vi "Plot_XY_data.vi"(0 "Channel Values":string[][](array[string]), 1 "Ordinate Strings":string[](array[string]), 2 "Swap color and symbol":i32, 3 "Error Bar Chs":i32[](array[numeric])=[11], 5 "Accept Array":bool[][](array[boolean]), 7 "Filter 1 Strings":string[](array[string]), 9 "Filter 2 Strings":string[](array[string]), 11 "Ordinate":i32[](array[numeric])=[11], 12 "Absisca":u16, 13 "Transpose":bool) -> (15 "Accept Array Out":bool[][](array[boolean]))   [LabVIEW 2015]
uses:
  Results_plotter_Global.vi
panel:
  out "Colour Array":u32[][](array[colorbox])=[[26112, 39168, 52224, 65280, 65433], [153, 13311, 26367, 52479, 65535], [16711680, 16724838, 16737894, 16737945, 16751103], [16776960, 16777062, 16777113, 16777164, 16777215], [65280, 65280, 65280, 65280, 65280], [65280, 65280, 65280, 65280, 102]]
  out "Point Choice":u8[](array[numeric])=[10, 1, 11, 15, 5, 13, 2, 14]
  in  "Index Filter2":i32
  in  "Index Filter1":i32
  in  "Index Ordinate":i32
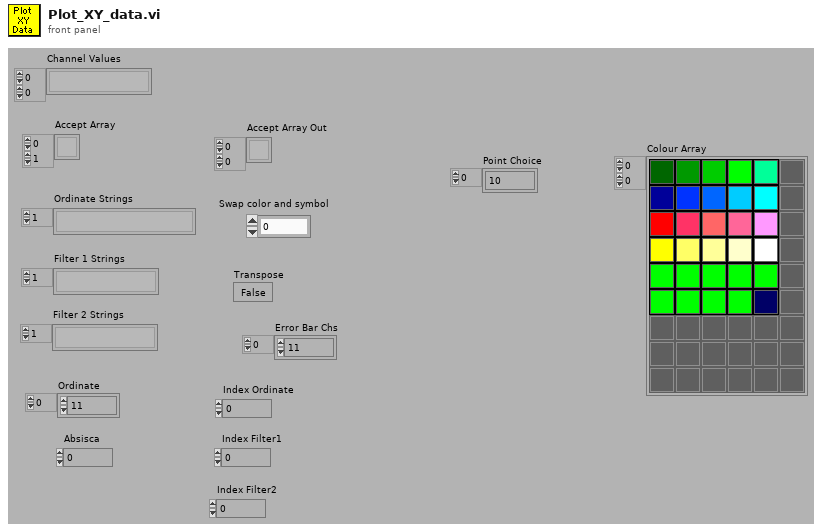
[diagram p1: front panel]
types:
  T1 = cluster{"Plot Color":u32, "Plot Interpolation":u8, "Point Style":u8, "Line Style":u8, "Fill/Pt. Color":u32, "Line Width":u8, "Bar Plot Style":u8, "Fill To":i16}
  T2 = cluster{"Averaged Values":dbl[], "Positions":dbl[]}[]
  T3 = cluster{"Plot Color":u32, "Plot Interpolation":u8, "Point Style":u8, "Line Style":u8, "Fill/Pt. Color":u32, "Line Width":u8, "Bar Plot Style":u8, "Fill To":i16}[]
  T4 = cluster{"Positions":dbl[], "Averaged Values":dbl[]}
  T5 = cluster{"Averaged Values":dbl[], "Positions":dbl[]}
  T6 = enum16{"Points", "StepLeft", "Line", "StepRight", "StepCentre", "StepEdge"}
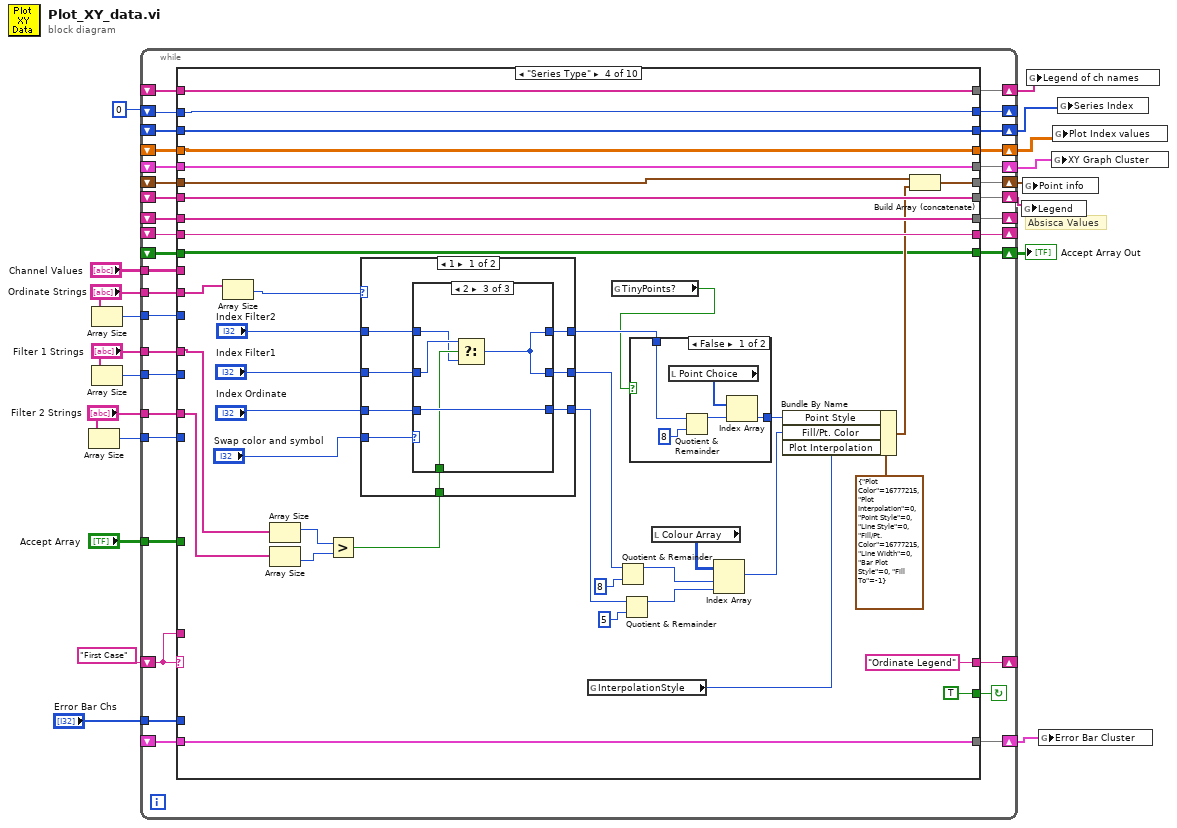
[diagram p0: block diagram]
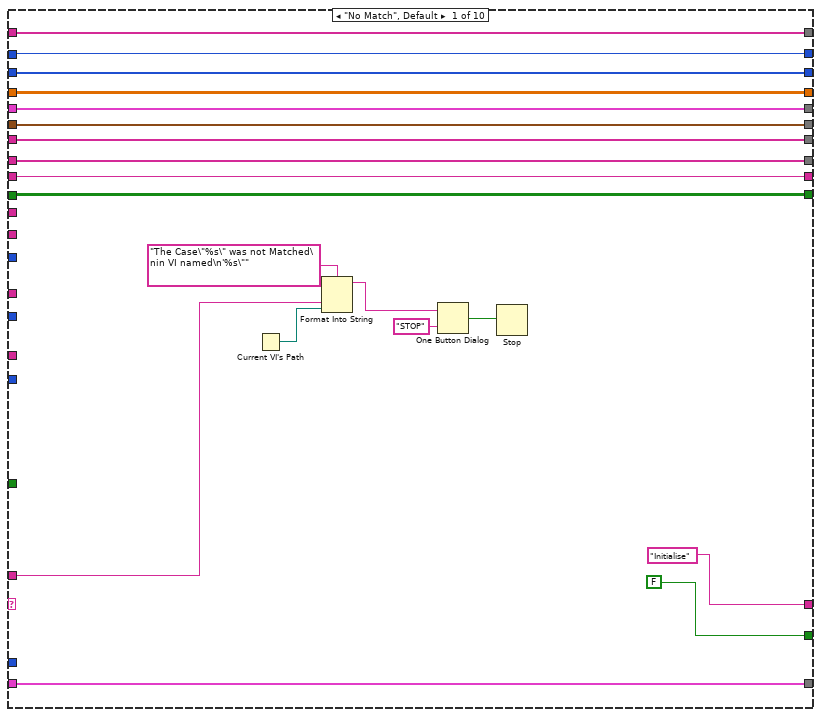
[diagram p2: hidden frame]
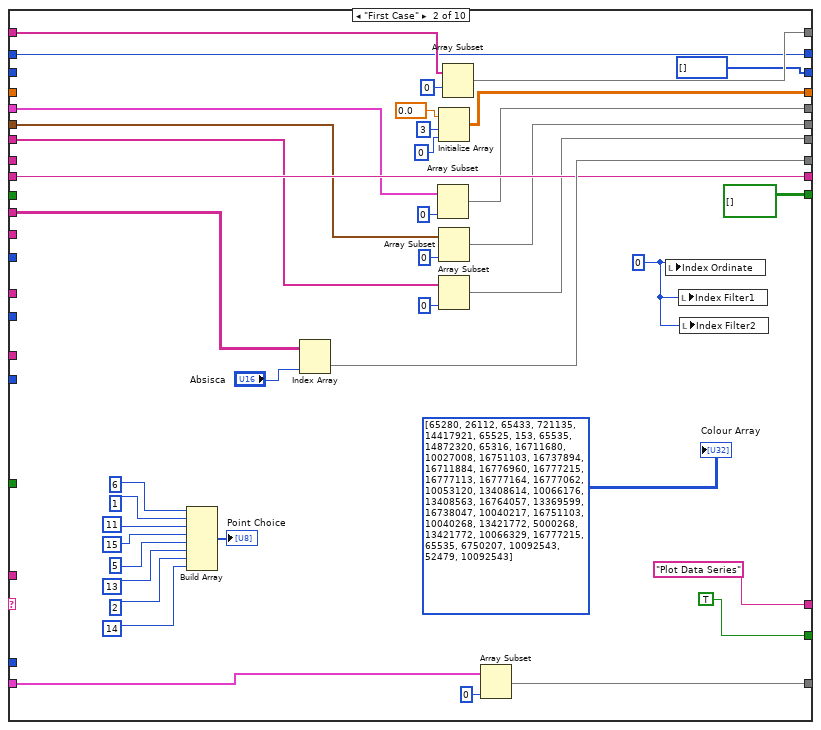
[diagram p3: hidden frame]
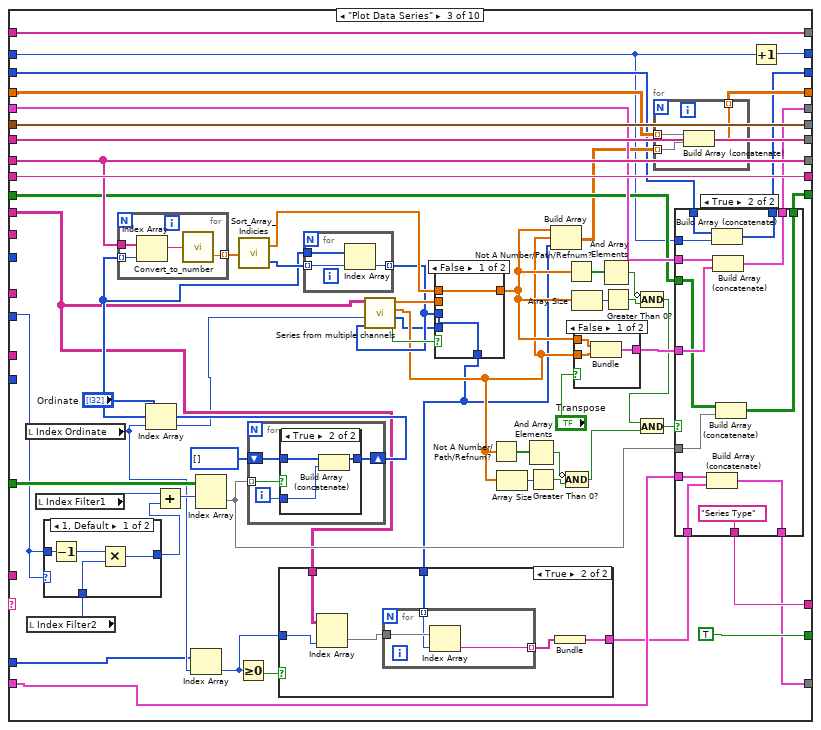
[diagram p4: hidden frame]
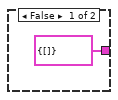
[diagram p6: hidden frame]
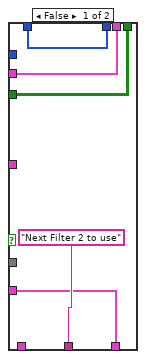
[diagram p8: hidden frame]
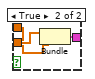
[diagram p9: hidden frame]
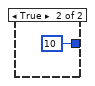
[diagram p11: hidden frame]
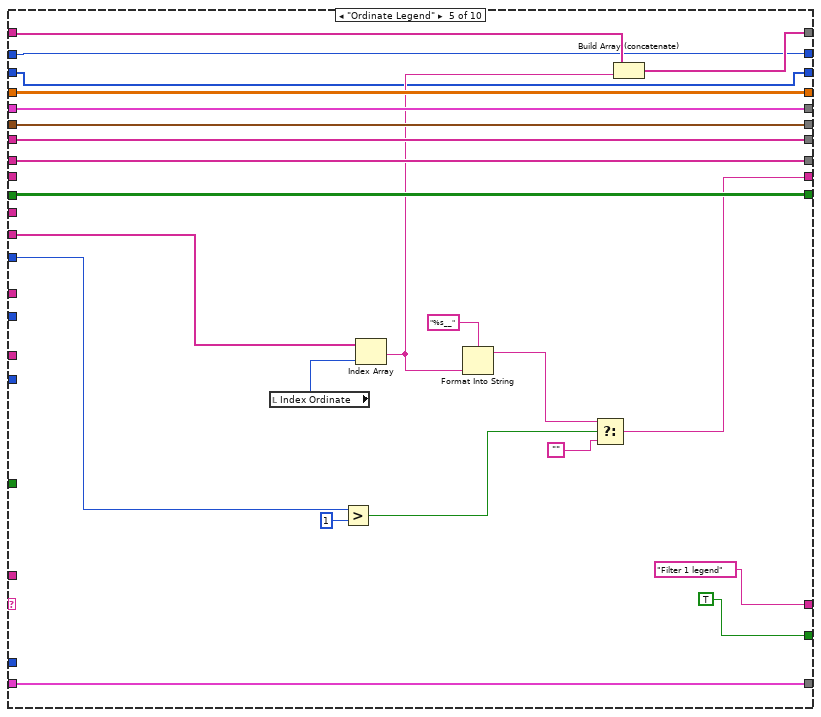
[diagram p20: hidden frame]
diagram:
  # "Absisca Values"
  n1 = Array Size(array="Filter 2 Strings") -> (size(s)=w12:i32)
  n2 = Array Size(array="Ordinate Strings") -> (size(s)=w13:i32)
  n3 = Array Size(array="Filter 1 Strings") -> (size(s)=w11:i32)
  n4 = while {
    shift-left: _ -> [w32]
    shift-right: [w31] -> w10
    tunnel: w11 -> [w33]
    tunnel: w12 -> [w34]
    tunnel: w13 -> [w35]
    tunnel: "Filter 1 Strings" -> [w36]
    tunnel: "Filter 2 Strings" -> [w37]
    tunnel: "Ordinate Strings" -> [w38]
    tunnel: "Accept Array" -> [w39]
    tunnel: "Channel Values" -> [w40]
    shift-left: _ -> [w41]
    shift-right: [w42] -> _
    shift-left: _ -> [w43]
    shift-right: [w44] -> _
    shift-left: _ -> [w46]
    shift-right: [w45] -> w7
    shift-left: _ -> [w48]
    shift-right: [w47] -> w8
    shift-left: _ -> [w50]
    shift-right: [w49] -> w6
    shift-left: "First Case" -> [w51]
    shift-right: [w52] -> _
    shift-right: [w29] -> w9
    shift-left: _ -> [w30]
    shift-right: [w28] -> w5
    shift-left: _ -> [w27]
    tunnel: "Error Bar Chs" -> [w26]
    shift-right: [w24] -> w3
    shift-left: _ -> [w25]
    shift-right: [w22] -> _
    shift-left: 0 -> [w23]
    shift-right: [w20] -> w1
    shift-left: _ -> [w21]
    stop <- w53 continue-if-true
    n5 = case shown="\"Series Type\"" w51 {
      tunnel: [FALSE TRUE TRUE TRUE TRUE TRUE TRUE TRUE TRUE w473] -> w53
      tunnel: ["Initialise" "Plot Data Series" w157 "Ordinate Legend" "Filter 1 legend" "Filter 2 Legend" "Next Filter 2 to use" w425 w449 w474] -> w52
      tunnel: w51 -> [w67 _ _ _ _ _ _ _ _ _]
      tunnel: w50 -> [w64 w95 w159 w269 w342 w359 w396 w435 w459 w484]
      tunnel: [w64 w94 w158 w269 w342 w359 w396 w435 w459 w484] -> w49
      tunnel: w48 -> [w63 w90 w170 w260 w339 w356 w394 w434 w458 w483]
      tunnel: [w63 w89 w170 w258 w339 w356 w394 w434 w458 w483] -> w47
      tunnel: w46 -> [w62 w88 w169 w268 w341 w358 w391 w433 w457 w482]
      tunnel: [w62 w87 w169 w268 w341 w358 w392 w433 w457 w482] -> w45
      tunnel: [w61 w107 w166 w267 w340 w357 w395 w432 w456 w481] -> w44
      tunnel: w43 -> [w61 _ w166 w267 w340 w357 w395 w432 w456 w481]
      tunnel: [w60 w96 w168 w266 w328 w355 w384 w431 w455 w480] -> w42
      tunnel: w41 -> [w60 w96 w168 w266 _ w352 w384 w431 w455 w480]
      tunnel: w40 -> [_ w108 w121 _ _ _ _ _ _ _]
      tunnel: w39 -> [_ _ w165 _ _ _ _ _ _ _]
      tunnel: w38 -> [_ _ _ w246 w336 _ _ _ _ _]
      tunnel: w37 -> [_ _ _ w243 _ _ w382 _ _ _]
      tunnel: w36 -> [_ _ _ w244 _ w353 _ _ _ _]
      tunnel: w35 -> [_ _ _ _ w338 _ _ _ _ w471]
      tunnel: w34 -> [_ _ _ _ _ _ w393 w421 _ _]
      tunnel: w33 -> [_ _ w150 _ _ w351 _ _ w445 _]
      tunnel: w32 -> [w59 _ w155 w256 w335 w350 w390 w424 w448 w472]
      tunnel: [w59 bool[][] [] w153 w256 w335 w350 w390 w424 w448 w472] -> w31
      tunnel: w30 -> [w58 _ w147 w255 w334 w349 w389 w423 w447 w470]
      tunnel: [w58 w84 w148 w255 w334 w349 w389 w423 w447 w470] -> w29
      tunnel: w27 -> [w57 w80 w146 w238 w325 w348 w388 w422 w446 w469]
      tunnel: [w57 w75 w146 w238 w326 w348 w388 w422 w446 w469] -> w28
      tunnel: w26 -> [_ _ w144 _ _ _ _ _ _ _]
      tunnel: w25 -> [w56 w77 w141 w237 w324 w347 w387 w420 w444 w468]
      tunnel: [w56 w76 w139 w237 w324 w347 w387 w420 w444 w468] -> w24
      tunnel: w23 -> [w55 w74 w122 w236 w323 w346 w386 w419 w443 w467]
      tunnel: [w55 w74 w125 w236 w323 w346 w386 w419 w443 w467] -> w22
      tunnel: w21 -> [w54 _ w124 w235 w322 w345 w385 w418 w442 w466]
      tunnel: [w54 i32[] [] w123 w235 w322 w345 w385 w418 w442 w466] -> w20
      frame "No Match", Default {
        n6 = Current VI's Path() -> (path=w66:path)
        n7 = Format Into String(format string="The Case\"%s\" was not Matched\nin VI named\n'%s\"" ("Format String"), w67, w66) -> (resulting string=w70:string)  [unwired: 2 in, 1 out]
        n8 = One Button Dialog(message=w70, button name ("OK")="STOP") -> (true=w68:bool)
        n9 = Stop(stop? (T)=w68) -> ()
      }
      frame "First Case" {
        w106 = 0
        n10 = Build Array(u8 6 ("Write Attribute"), u8 1 ("Write Attribute"), u8 11 ("Write Attribute"), u8 15 ("Write Attribute"), u8 5 ("Write Attribute"), u8 13 ("Write Attribute"), u8 2 ("Write Attribute"), u8 14 ("Write Attribute")) -> (→"Point Choice":u8[])
        n11 = Index Array(array=w108, index (col)="Absisca") -> (element=w107:string[])  [unwired: 1 in]
        n12 = Array Subset(array=w95, length=0 ("Array Length")) -> (w94:T2)  [unwired: 1 in]
        n13 = Initialize Array(0.0 ("element"), 3 ("dimension size"), 0 ("dimension size")) -> (w84:dbl[][])
        n14 = Array Subset(array=w90, length=0 ("Array Length")) -> (w89:T3)  [unwired: 1 in]
        n15 = Array Subset(array=w88, length=0 ("Array Length")) -> (w87:string[])  [unwired: 1 in]
        n16 = Array Subset(array=w80, length=0) -> (w75:string[])  [unwired: 1 in]
        n17 = Array Subset(array=w77, length=0 ("Array Length")) -> (w76:cluster{string[]}[])  [unwired: 1 in]
        n18 = local write "Index Ordinate"(w106) -> ()
        n19 = local write "Index Filter1"(w106) -> ()
        n20 = local write "Index Filter2"(w106) -> ()
        "Colour Array" <- u32[][] [[65280, 26112, 65433, 721135, 14417921], [65525, 153, 65535, 14872320, 65316], [16711680, 10027008, 16751103, 16737894, 16711884], [16776960, 16777215, 16777113, 16777164, 16777062], [10053120, 13408614, 10066176, 13408563, 16764057], [13369599, 16738047, 10040217, 16751103, 10040268], [13421772, 5000268, 13421772, 10066329, 16777215], [65535, 6750207, 10092543, 52479, 10092543]] ("Output Array 2")
      }
      frame "Plot Data Series" {
        n21 = local read "Index Ordinate"() -> (w145:i32)
        n22 = local read "Index Filter2"() -> (w152:i32)
        n23 = local read "Index Filter1"() -> (w164:i32)
        n24 = case shown="1, Default" w150 {
          tunnel: w152 -> [w195 w196]
          tunnel: w150 -> [w194 _]
          tunnel: [w193 w196] -> w151
          frame 1, Default {
            n25 = Decrement(x=w194) -> (x-1=w192:i32)
            n26 = Multiply(x=w192, y=w195) -> (x*y=w193:i32)
          }
          frame 0 {
          }
        }
        n27 = Index Array(array="Ordinate", index=w145) -> (element=w120:i32)
        n28 = Add(x=w164, y=w151) -> (x+y=w163:i32)
        n29 = Index Array(array=w144, index=w145) -> (element=w142:i32)
        n30 = Index Array(array=w165, index (row)=w163) -> (element=w154:bool[])  [unwired: 1 in]
        n31 = Greater Or Equal To 0?(x=w142) -> (x >= 0?=w143:bool)
        n32 = for {
          shift-right: [w226] -> w136
          shift-left: i32[] [] -> [w227]
          tunnel: w154 -> [w225] mode=indexing
          i -> [w228]
          n33 = case shown="True" w225 {
            tunnel: w228 -> [_ w232]
            tunnel: w227 -> [w229 w231]
            tunnel: [w229 w230] -> w226
            frame False {
            }
            frame True {
              n34 = Build Array (concatenate)(w231, w232) -> (w230:i32[])
            }
          }
        }
        n35 = for {
          tunnel: w166 -> [w218]
          tunnel: [w216] -> w138 mode=indexing
          tunnel: w136 -> [w217] mode=indexing
          n36 = Index Array(array=w218, index=w217) -> (element=w215:string)
          n37 = call "Convert_to_number.vi"("string"=w215) -> ("Number"=w216:dbl)  [unwired: 1 out]
        }
        n38 = call "Sort_Array_Indicies.vi"("unsorted array"=w138) -> ("sorted array"=w118:dbl[], "Sort Index"=w137:i32[])
        n39 = for {
          tunnel: w137 -> [w178] mode=indexing
          tunnel: w136 -> [w177]
          tunnel: [w176] -> w115 mode=indexing
          n40 = Index Array(array=w177, index=w178) -> (element=w176:i32)
        }
        n41 = call "Series from multiple channels.vi"("Row Numbers"=w115, "Ordinate Index"=w120, "Channel Values"=w121) -> ("Plot?"=w119:bool, "Row Numbers Out"=w112:i32[], "Averaged Values"=w114:dbl[], "Positions"=w116:dbl[])  [unwired: 5 in]
        n42 = case shown="False" w119 {
          tunnel: [w173 w175] -> w117
          tunnel: w118 -> [w173 _]
          tunnel: w116 -> [_ w175]
          tunnel: [w172 w174] -> w113
          tunnel: w115 -> [w172 _]
          tunnel: w112 -> [_ w174]
          frame False {
          }
          frame True {
          }
        }
        n43 = case shown="True" w143 {
          tunnel: w121 -> [_ w185]
          tunnel: w142 -> [_ w184]
          tunnel: w113 -> [_ w182]
          tunnel: [cluster{string[]} {[]} w181] -> w140
          frame False {
          }
          frame True {
            n44 = Index Array(array=w185, index (col)=w184) -> (element=w183:string[])  [unwired: 1 in]
            n45 = for {
              tunnel: w183 -> [w188]
              tunnel: w182 -> [w187] mode=indexing
              tunnel: [w186] -> w180 mode=indexing
              n46 = Index Array(array=w188, index=w187) -> (element=w186:string)
            }
            n47 = Bundle(w180) -> (w181:cluster{string[]})  [unwired: 1 in]
          }
        }
        n48 = Not A Number/Path/Refnum?(number/path/refnum=w114) -> (NaN/Path/Refnum?=w131:bool[])
        n49 = Array Size(array=w114) -> (size(s)=w132:i32)
        n50 = And Array Elements(Boolean array=w131) -> (logical AND=w129:bool)
        n51 = Greater Than 0?(x=w132) -> (x > 0?=w130:bool)
        n52 = Build Array(w117, w114, w113) -> (w149:dbl[][])
        n53 = Not A Number/Path/Refnum?(number/path/refnum=w117) -> (NaN/Path/Refnum?=w135:bool[])
        n54 = Compound Arithmetic op=AND(invert w129, w130) -> (w126:bool)
        n55 = Array Size(array=w117) -> (size(s)=w161:i32)
        n56 = case shown="False" "Transpose" {
          tunnel: w117 -> [w221 w222]
          tunnel: [w220 w224] -> w160
          tunnel: w114 -> [w219 w223]
          frame False {
            n57 = Bundle("Positions"=w221, "Averaged Values"=w219) -> (w220:T4)  [unwired: 1 out]
          }
          frame True {
            n58 = Bundle("Averaged Values"=w223, "Positions"=w222) -> (w224:T5)  [unwired: 1 out]
          }
        }
        n59 = And Array Elements(Boolean array=w135) -> (logical AND=w133:bool)
        n60 = Greater Than 0?(x=w161) -> (x > 0?=w134:bool)
        n61 = Compound Arithmetic op=AND(invert w133, w134) -> (w127:bool)
        n62 = And(x=w127, y=w126) -> (x .and. y?=w128:bool)
        n63 = for {
          tunnel: w147 -> [w189] mode=indexing
          tunnel: w149 -> [w191] mode=indexing
          tunnel: [w190] -> w148 mode=indexing
          n64 = Build Array (concatenate)(w189, w191) -> (w190:dbl[])
        }
        n65 = case shown="True" w128 {
          tunnel: w160 -> [_ w214]
          tunnel: w159 -> [w200 w213]
          tunnel: [w200 w205] -> w158
          tunnel: ["Next Filter 2 to use" "Series Type"] -> w157
          tunnel: w155 -> [w199 w211]
          tunnel: w154 -> [_ w210]
          tunnel: [w199 w209] -> w153
          tunnel: w141 -> [w198 w208]
          tunnel: w140 -> [_ w207]
          tunnel: [w198 w206] -> w139
          tunnel: w124 -> [w197 w204]
          tunnel: [w197 w203] -> w123
          tunnel: w122 -> [_ w202]
          frame False {
          }
          frame True {
            n66 = Build Array (concatenate)(w208, w207) -> (w206:cluster{string[]}[])
            n67 = Build Array (concatenate)(w204, w202) -> (w203:i32[])
            n68 = Build Array (concatenate)(w213, w214) -> (w205:T2)
            n69 = Build Array (concatenate)(w211, w210) -> (w209:bool[][])
          }
        }
        n70 = Increment(x=w122) -> (x+1=w125:i32)
      }
      frame "Series Type" {
        n71 = Array Size(array=w246) -> (size(s)=w245:i32)
        n72 = Array Size(array=w244) -> (size(s)=w242:i32)
        n73 = Array Size(array=w243) -> (size(s)=w241:i32)
        n74 = Greater?(x=w242, y=w241) -> (0:w240:bool)
        n75 = case shown="1" w245 {
          tunnel: [w285 w303] -> w239
          tunnel: "Index Filter2" -> [w284 w302]
          tunnel: [w283 w301] -> w251
          tunnel: "Index Filter1" -> [w282 w300]
          tunnel: "Index Ordinate" -> [w281 w299]
          tunnel: [w280 w298] -> w248
          tunnel: "Swap color and symbol" -> [w279 w297]
          tunnel: w240 -> [w278 _]
          frame 1 {
            n76 = case shown="2" w279 {
              tunnel: [w288 w290 w292] -> w285
              tunnel: w284 -> [w288 w289 w293]
              tunnel: [w287 w289 w292] -> w283
              tunnel: w282 -> [w287 w290 w294]
              tunnel: w281 -> [w286 w291 w296]
              tunnel: [w286 w291 w296] -> w280
              tunnel: w278 -> [_ _ w295]
              frame 0, Default {
              }
              frame 1 {
              }
              frame 2 {
                n77 = Select(t=w294, s=w295, f=w293) -> (s? t:f=w292:i32)
              }
            }
          }
          frame 2, Default {
            n78 = case shown="4" w297 {
              tunnel: [w306 w308 w310 w314 w318 w321] -> w303
              tunnel: w302 -> [w306 w307 w310 w313 w316 w320]
              tunnel: [w305 w307 w312 w315 w317 w320] -> w301
              tunnel: w300 -> [w305 w308 w311 w314 w317 w319]
              tunnel: w299 -> [w304 w309 w312 w315 w318 w321]
              tunnel: [w304 w309 w311 w313 w316 w319] -> w298
              frame 0, Default {
              }
              frame 1 {
              }
              frame 2 {
              }
              frame 3 {
              }
              frame 4 {
              }
              frame 5 {
              }
            }
          }
        }
        n79 = global read "Results_plotter_Global.vi" "InterpolationStyle"() -> (w233:T6)
        n80 = global read "Results_plotter_Global.vi" "TinyPoints?"() -> (w234:bool)
        n81 = Quotient & Remainder(x=w251, y=8) -> (x-y*floor(x/y)=w254:i32)  [unwired: 1 out]
        n82 = Quotient & Remainder(x=w248, y=5) -> (x-y*floor(x/y)=w253:i32)  [unwired: 1 out]
        n83 = case shown="False" w234 {
          tunnel: [w275 u8 10 ("Write Attribute")] -> w262
          tunnel: w239 -> [w273 _]
          frame False {
            n84 = local read "Point Choice"() -> (w276:u8[])
            n85 = Quotient & Remainder(x=w273, y=8) -> (x-y*floor(x/y)=w272:i32)  [unwired: 1 out]
            n86 = Index Array(array=w276, index=w272) -> (element=w275:u8)
          }
          frame True {
          }
        }
        n87 = local read "Colour Array"() -> (w263:u32[][])
        n88 = Index Array(array=w263, index (row)=w254, index (col)=w253) -> (element=w261:u32)
        n89 = Bundle By Name(cluster=T1 {"Plot Color"=16777215, "Plot Interpolation"=0, "Point Style"=0, "Line Style"=0, "Fill/Pt. Color"=16777215, "Line Width"=0, "Bar Plot Style"=0, "Fill To"=-1} ("Read Attribute"), "Point Style"=w262, "Fill/Pt. Color"=w261, "Plot Interpolation"=w233) -> (w259:T1)
        n90 = Build Array (concatenate)(w260, w259) -> (w258:T3)
      }
      frame "Ordinate Legend" {
        n91 = local read "Index Ordinate"() -> (w332:i32)
        n92 = Greater?(x=w338, y=1) -> (0:w331:bool)
        n93 = Index Array(array=w336, index=w332) -> (element=w327:string)
        n94 = Format Into String(format string="%s__" ("Format String"), w327) -> (resulting string=w330:string)  [unwired: 2 in, 1 out]
        n95 = Select(t=w330, s=w331, f="") -> (s? t:f=w328:string)
        n96 = Build Array (concatenate)(w325, w327) -> (w326:string[])
      }
      frame "Filter 1 legend" {
        n97 = Greater Than 0?(x=w351) -> (x > 0?=w354:bool)
        n98 = case shown="True" w354 {
          tunnel: [w362 w372] -> w355
          tunnel: w353 -> [_ w371]
          tunnel: w352 -> [w362 w374]
          frame False {
          }
          frame True {
            n99 = local read "Index Filter1"() -> (w376:i32)
            n100 = Index Array(array=w371, index=0 ("Index")) -> (element=w369:string)
            n101 = Increment(x=w376) -> (x+1=w370:i32)
            n102 = Index Array(array=w371, index=w370) -> (element=w375:string)
            n103 = Match Pattern(string=w375, regular expression=" (") -> (before substring=w365:string)  [unwired: 4 out]
            n104 = String Subset(string=w365, length (rest)=15 ("length (rest)")) -> (substring=w363:string)  [unwired: 1 in]
            n105 = Match Pattern(string=w363, regular expression="=") -> (offset past match=w367:i32)  [unwired: 1 in, 3 out]
            n106 = Less Than 0?(x=w367) -> (x < 0?=w366:bool)
            n107 = case shown="False" w366 {
              tunnel: ["%s=%s__" ("Format String") "%s %s__" ("Format String")] -> w373
              frame True {
              }
              frame False {
              }
            }
            n108 = Format Into String(format string=w373, initial string=w374, w369, w365) -> (resulting string=w372:string)  [unwired: 1 in, 1 out]
          }
        }
      }
      frame "Filter 2 Legend" {
        n109 = Greater Than 0?(x=w393) -> (x > 0?=w381:bool)
        n110 = case shown="True" w381 {
          tunnel: [w399 w410] -> w383
          tunnel: w382 -> [_ w409]
          tunnel: w384 -> [w399 w412]
          frame False {
          }
          frame True {
            n111 = local read "Index Filter2"() -> (w403:i32)
            n112 = Index Array(array=w409, index=0 ("Index")) -> (element=w407:string)
            n113 = Increment(x=w403) -> (x+1=w408:i32)
            n114 = Index Array(array=w409, index=w408) -> (element=w413:string)
            n115 = Match Pattern(string=w413, regular expression=" (") -> (before substring=w401:string)  [unwired: 4 out]
            n116 = String Subset(string=w401, length (rest)=15 ("length (rest)")) -> (substring=w400:string)  [unwired: 1 in]
            n117 = Match Pattern(string=w400, regular expression="=") -> (offset past match=w405:i32)  [unwired: 1 in, 3 out]
            n118 = Less Than 0?(x=w405) -> (x < 0?=w404:bool)
            n119 = case shown="True" w404 {
              tunnel: ["%s=%s__" ("Format String") "%s%s__" ("Format String")] -> w411
              frame True {
              }
              frame False {
              }
            }
            n120 = Format Into String(format string=w411, initial string=w412, w407, w401) -> (resulting string=w410:string)  [unwired: 1 in, 1 out]
          }
        }
        n121 = Build Array (concatenate)(w391, w383) -> (w392:string[])
      }
      frame "Next Filter 2 to use" {
        n122 = local read "Index Filter2"() -> (w427:i32)
        n123 = Add(x=w427, y=2 ("x")) -> (x+y=w430:i32)
        n124 = Less?(x=w430, y=w421) -> (x < y?=w429:bool)
        n125 = case shown="False" w429 {
          tunnel: w427 -> [_ w441]
          tunnel: [0 w440] -> w426
          tunnel: ["Next Filter 1 to use" "Plot Data Series"] -> w425
          frame False {
          }
          frame True {
            n126 = Increment(x=w441) -> (x+1=w440:i32)
          }
        }
        n127 = local write "Index Filter2"(w426) -> ()
      }
      frame "Next Filter 1 to use" {
        n128 = local read "Index Filter1"() -> (w451:i32)
        n129 = Add(x=w451, y=2 ("x")) -> (x+y=w454:i32)
        n130 = Less?(x=w454, y=w445) -> (x < y?=w453:bool)
        n131 = case shown="False" w453 {
          tunnel: w451 -> [_ w465]
          tunnel: [0 w464] -> w450
          tunnel: ["Next Ordinate" "Plot Data Series"] -> w449
          frame False {
          }
          frame True {
            n132 = Increment(x=w465) -> (x+1=w464:i32)
          }
        }
        n133 = local write "Index Filter1"(w450) -> ()
      }
      frame "Next Ordinate" {
        n134 = local read "Index Ordinate"() -> (w476:i32)
        n135 = Add(x=w476, y=1 ("x")) -> (x+y=w479:i32)
        n136 = Less?(x=w479, y=w471) -> (x < y?=w478:bool)
        n137 = case shown="False" w478 {
          tunnel: w476 -> [_ w491]
          tunnel: [0 w490] -> w475
          tunnel: ["End" "Plot Data Series"] -> w474
          tunnel: [FALSE TRUE] -> w473
          frame False {
          }
          frame True {
            n138 = Increment(x=w491) -> (x+1=w490:i32)
          }
        }
        n139 = local write "Index Ordinate"(w475) -> ()
      }
    }
  }
  "Accept Array Out" <- w10
  n140 = global write "Results_plotter_Global.vi" "Legend"(w7) -> ()
  n141 = global write "Results_plotter_Global.vi" "Point info"(w8) -> ()
  n142 = global write "Results_plotter_Global.vi" "Legend of ch names"(w5) -> ()
  n143 = global write "Results_plotter_Global.vi" "Error Bar Cluster"(w3) -> ()
  n144 = global write "Results_plotter_Global.vi" "XY Graph Cluster"(w6) -> ()
  n145 = global write "Results_plotter_Global.vi" "Plot Index values"(w9) -> ()
  n146 = global write "Results_plotter_Global.vi" "Series Index"(w1) -> ()
